vi "Sub_Electrical_Noise_Analysis-Excel-2.vi"(11 "iteration(0)":i32) -> (3 "Output":string[](array[string]))   [LabVIEW 2015]
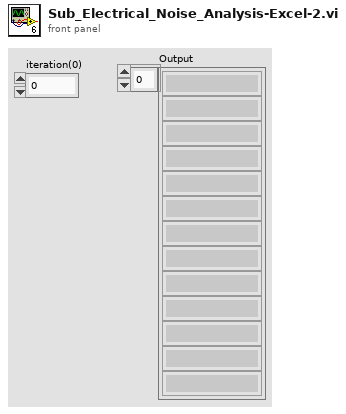
[diagram p1: front panel]
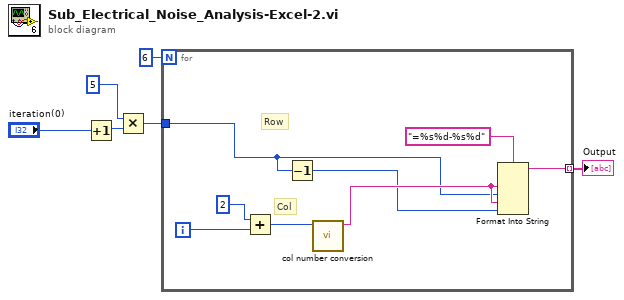
[diagram p0: block diagram]
diagram:
  n1 = Increment(x="iteration(0)") -> (x+1=w5:i32)
  n2 = Multiply(x=5, y=w5) -> (x*y=w3:i32)
  n3 = for {
    N: 6 -> [_]
    tunnel: w3 -> [w7]
    tunnel: [w8] -> w1 mode=indexing
    i -> [w12]
    # "Row"
    # "Col"
    n4 = Add(x=2, y=w12) -> (x+y=w13:i32)
    n5 = Decrement(x=w7) -> (x-1=w9:i32)
    n6 = call "col number conversion.vi"("Col Number"=w13) -> ("Excel Col Number"=w10:string)  [unwired: 10 in]
    n7 = Format Into String(format string="=%s%d-%s%d" ("포맷 문자열"), w10, w7, w10, w9) -> (resulting string=w8:string)  [unwired: 2 in, 1 out]
  }
  "Output" <- w1
